vi "Generate Start Measurement Command.vi"(0 "Sensor Address In":string="a", 1 "CRC (False)":bool, 2 "Parameter (0)":i32(ring) items=["0", "1", "2", "3", "4", "5", "6", "7", "8", "9"], 7 "Measurement Type In (Normal)":i32(ring) items=["Normal", "Concurrent", "Continuous"], 11 "Error In (No Error)":errorcluster) -> (4 "Command":string, 15 "Error Out":errorcluster)   [LabVIEW 2016, in "SDI-12.lvlib"]
doc: "Generates a Normal or Concurrent Start Measurement Command, depending on the settings passed to the controls.\n\nStart Measurement aM!\nStart Measurement and Request CRC aMC!\nAdditional Measurements aM1! through aM9!\nAdditional Measurements and Request CRC aMC1! through aMC9!\nStart Concurrent Measurement aC!\nStart Concurrent Measurement and Request CRC aCC!\nAdditional Concurrent Measurements aC1! through aC9!\nAdditional Concurrent Measurements and Request CRC aCC1! through aCC9!\n\n\nNOTE: Continuous Measurements are continuously acquiring data, and should not be sent a Start Measurement Command."
uses:
  SDI-12.lvlib
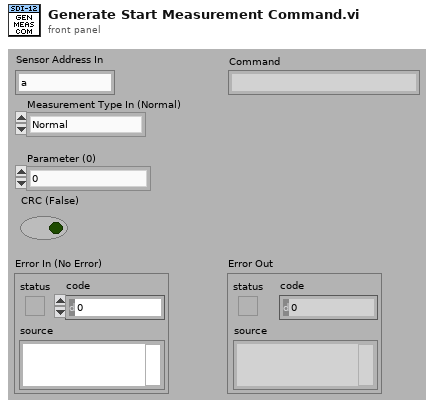
[diagram p1: front panel]
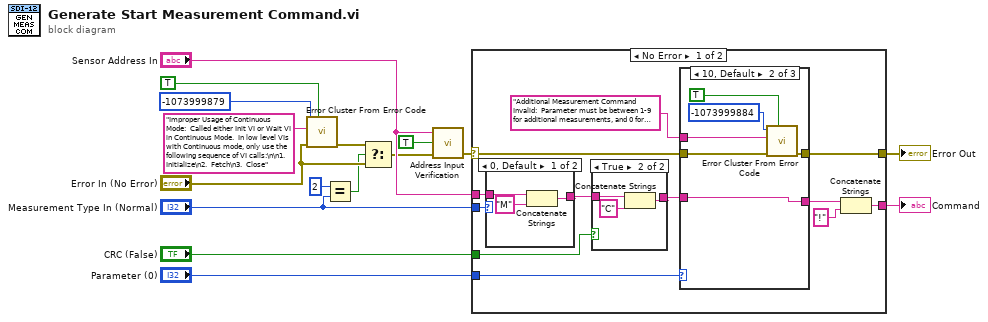
[diagram p0: block diagram]
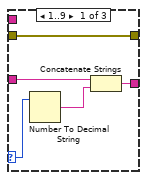
[diagram p3: hidden frame]
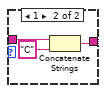
[diagram p5: hidden frame]
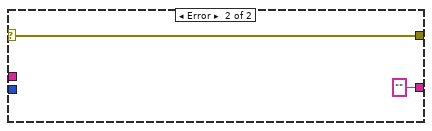
[diagram p6: hidden frame]
diagram:
  n1 = call <vilib>:"Error Cluster From Error Code.vi"("show call chain? (False)"=TRUE ("Error?"), "error in (no error)"="Error In (No Error)", "error message (\"\")"="Improper Usage of Continuous Mode:  Called either Init VI or Wait VI in Continuous Mode.  In low level VIs with Continuous mode, only use the following sequence of VI calls:\n\n1.  Initialize\n2.  Fetch\n3.  Close" ("error message (\"\")"), "error code (0)"=-1073999879 ("error code")) -> ("error out"=w7:errorcluster)  [unwired: 5 in]
  n2 = Equal?(x=2, y="Measurement Type In (Normal)") -> (x = y?=w1:bool)
  n3 = Select(t=w7, s=w1, f="Error In (No Error)") -> (s? t:f=w4:errorcluster)
  n4 = call "Address Input Verification.vi"("Error In (No Error)"=w4, "Error if Bad? (True)"=TRUE ("error if bad? (True)"), "Sensor Address In (a)"="Sensor Address In") -> ("Error Out"=w14:errorcluster)  [unwired: 1 in, 1 out]
  n5 = case shown="No Error" w14 {
    selector: w14 -> [w20 w53]
    tunnel: "Sensor Address In" -> [w28 _]
    tunnel: [w19 w53] -> w16
    tunnel: "Measurement Type In (Normal)" -> [w24 _]
    tunnel: "CRC (False)" -> [w22 _]
    tunnel: "Parameter (0)" -> [w23 _]
    tunnel: [w21 ""] -> w13
    frame No Error {
      n6 = case shown="0, Default" w24 {
        tunnel: w28 -> [w47 w51]
        tunnel: [w46 w49] -> w18
        frame 0, Default {
          n7 = Concatenate Strings(w47, "M" ("string")) -> (w46:string)
        }
        frame 1 {
          n8 = Concatenate Strings(w51, "C" ("string")) -> (w49:string)
        }
      }
      n9 = case shown="True" w22 {
        tunnel: w18 -> [w29 w32]
        tunnel: [w29 w30] -> w27
        frame False {
        }
        frame True {
          n10 = Concatenate Strings(w32, "C" ("string")) -> (w30:string)
        }
      }
      n11 = case shown="10, Default" w23 {
        selector: w23 -> [w37 _ _]
        tunnel: w27 -> [w35 w41 w45]
        tunnel: [w34 w41 w45] -> w26
        tunnel: w20 -> [w33 w40 w44]
        tunnel: [w33 w39 w44] -> w19
        tunnel: "Additional Measurement Command Invalid:  Parameter must be between 1-9 for additional measurements, and 0 for default measurements. " ("error message (\"\")") -> [_ w38 _]
        frame 1..9 {
          n12 = Number To Decimal String(number=w37) -> (decimal integer string=w36:string)  [unwired: 1 in]
          n13 = Concatenate Strings(w35, w36) -> (w34:string)
        }
        frame 10, Default {
          n14 = call <vilib>:"Error Cluster From Error Code.vi"("show call chain? (False)"=TRUE, "error in (no error)"=w40, "error message (\"\")"=w38, "error code (0)"=-1073999884 ("error code")) -> ("error out"=w39:errorcluster)  [unwired: 5 in]
        }
        frame 0 {
        }
      }
      n15 = Concatenate Strings(w26, "!" ("string")) -> (w21:string)
    }
    frame Error {
    }
  }
  "Error Out" <- w16
  "Command" <- w13
